vi "labviewRT_sm_example.vi"() -> ()   [LabVIEW 2020]
uses:
  lib/labviewRT-EPICS/sm bool read and increment.vi
  lib/labviewRT-EPICS/sm double read and increment.vi
  lib/labviewRT-EPICS/sm single read and increment.vi
  lib/labviewRT-EPICS/sm i64 read and increment.vi
  lib/labviewRT-EPICS/sm i32 read and increment.vi
  lib/labviewRT-EPICS/sm i16 read and increment.vi
  lib/labviewRT-EPICS/sm i8 read and increment.vi
  lib/labviewRT-EPICS/sm u64 read and increment.vi
  lib/labviewRT-EPICS/sm u32 read and increment.vi
  lib/labviewRT-EPICS/sm u16 read and increment.vi
  lib/labviewRT-EPICS/sm u8 read and increment.vi
  lib/labviewRT-EPICS/sm double write and increment.vi
  lib/labviewRT-EPICS/sm single write and increment.vi
  lib/labviewRT-EPICS/sm i64 write and increment.vi
  lib/labviewRT-EPICS/sm i32 write and increment.vi
  lib/labviewRT-EPICS/sm i16 write and increment.vi
  lib/labviewRT-EPICS/sm i8 write and increment.vi
  lib/labviewRT-EPICS/sm u64 write and increment.vi
  lib/labviewRT-EPICS/sm u32 write and increment.vi
  lib/labviewRT-EPICS/sm u16 write and increment.vi
  lib/labviewRT-EPICS/sm u8 write and increment.vi
  lib/labviewRT-EPICS/sm bool write and increment.vi
  lib/labviewRT-EPICS/linuxSharedMemory.lvlib
panel:
  in  "Boolean in":bool
  in  "U8":u8
  in  "U16":u16
  in  "U32":u32
  in  "U64":u64
  in  "I8":i8
  in  "I16":i16
  in  "I32":i32
  in  "I64":i64
  in  "Single":sgl format="%#_64g"
  in  "double":dbl format="%#_64g"
  out "U8":u8
  out "U16":u16
  out "U32":u32
  out "U64":u64
  out "I8":i8
  out "I16":i16
  out "I32":i32
  out "I64":i64
  out "Single":sgl format="%#_64g"
  out "double":dbl format="%#_64g"
  out "Boolean":bool
  in  "stop":bool
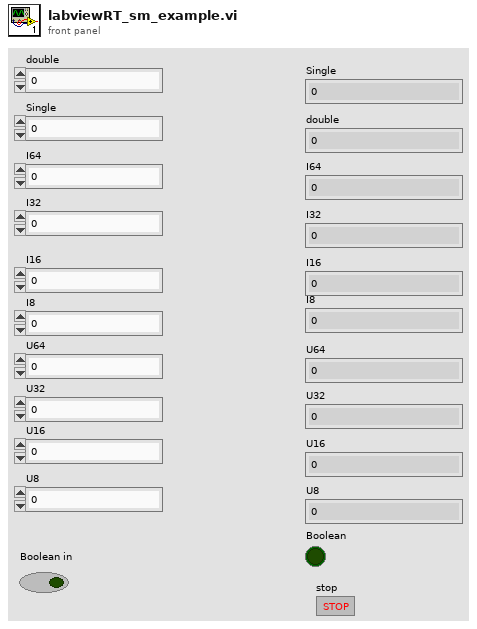
[diagram p1: front panel]
types:
  T1 = typedef "linuxSharedMemory.lvlib/sm_cluster.ctl" = cluster{"rt list":string, "error (no error)":errorcluster, "pointer":u64, "upper bound ptr":u64}
  T2 = typedef "Linux RT IPC.Shared Memory.lvlib/reference.ctl" = refnum<data-value>
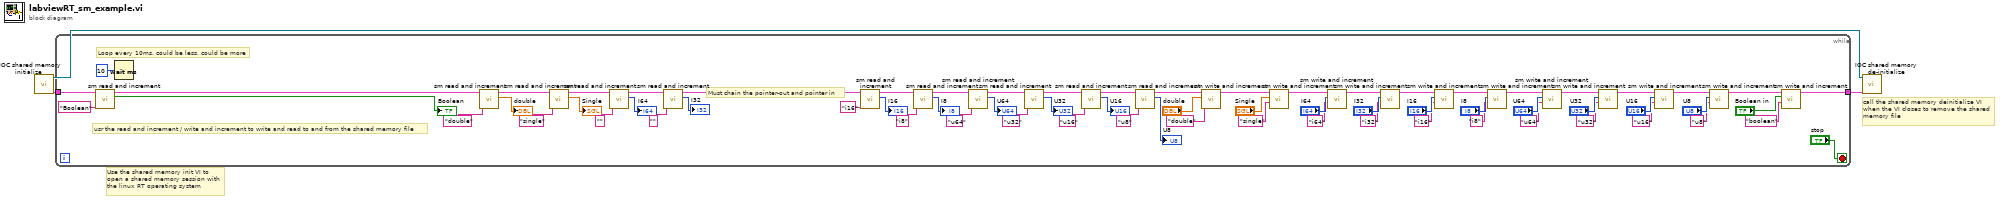
[diagram p0: block diagram]
diagram:
  # "call the shared memory deinitialize VI \nwhen the VI closes to remove the shared\nmemory file"
  # "Use the shared memory init VI to \nopen a shared memory session with\nthe linux RT operating system"
  n1 = call "IOC shared memory initialize.vi"() -> ("Shared memory cluster"=w2:T1, "shared memory class"=w3:T2)  [unwired: 10 in]
  n2 = while {
    tunnel: w2 -> [w27]
    tunnel: [w26] -> w1
    stop <- "stop" stop-if-true
    # "usr the read and increment / write and increment to write and read to and from the shared memory file"
    # "Must chain the pointer-out and pointer in"
    # "Loop every 10ms, could be less, could be more"
    n3 = call-poly "sm read and increment.vi"("Identifier"="Boolean", "Shared memory cluster input"=w27) -> ("Bool out"=→"Boolean":bool, "Shared memory cluster output"=w70:T1)  [unwired: 8 in]
    n4 = Wait (ms)(milliseconds to wait=10) -> ()  [unwired: 1 out]
    n5 = call-poly "sm read and increment.vi"("Identifier"="double", "Shared memory cluster input"=w70) -> ("Value out"=→"double":dbl, "Shared memory cluster output"=w69:T1)  [unwired: 8 in]
    n6 = call-poly "sm read and increment.vi"("Identifier"="single", "Shared memory cluster input"=w69) -> ("Value out"=→"Single":sgl, "Shared memory cluster output"=w68:T1)  [unwired: 8 in]
    n7 = call-poly "sm read and increment.vi"("Identifier"="", "Shared memory cluster input"=w68) -> ("Value out"=→"I64":i64, "Shared memory cluster output"=w67:T1)  [unwired: 8 in]
    n8 = call-poly "sm read and increment.vi"("Identifier"="", "Shared memory cluster input"=w67) -> ("Value out"=→"I32":i32, "Shared memory cluster output"=w66:T1)  [unwired: 8 in]
    n9 = call-poly "sm read and increment.vi"("Identifier"="i16", "Shared memory cluster input"=w66) -> ("Value out"=→"I16":i16, "Shared memory cluster output"=w65:T1)  [unwired: 8 in]
    n10 = call-poly "sm read and increment.vi"("Identifier"="i8", "Shared memory cluster input"=w65) -> ("Value out"=→"I8":i8, "Shared memory cluster output"=w64:T1)  [unwired: 8 in]
    n11 = call-poly "sm read and increment.vi"("Identifier"="u64", "Shared memory cluster input"=w64) -> ("Value out"=→"U64":u64, "Shared memory cluster output"=w63:T1)  [unwired: 8 in]
    n12 = call-poly "sm read and increment.vi"("Identifier"="u32", "Shared memory cluster input"=w63) -> ("Value out"=→"U32":u32, "Shared memory cluster output"=w61:T1)  [unwired: 8 in]
    n13 = call-poly "sm read and increment.vi"("Identifier"="u16", "Shared memory cluster input"=w61) -> ("Value out"=→"U16":u16, "Shared memory cluster output"=w62:T1)  [unwired: 8 in]
    n14 = call-poly "sm read and increment.vi"("Identifier"="u8", "Shared memory cluster input"=w62) -> ("Value out"=→"U8":u8, "Shared memory cluster output"=w48:T1)  [unwired: 8 in]
    n15 = call-poly "sm write and increment.vi"("Identifier"="double", "value in"="double", "Shared memory cluster input"=w48) -> ("Shared memory cluster output"=w47:T1)  [unwired: 8 in]
    n16 = call-poly "sm write and increment.vi"("Identifier"="single", "value in"="Single", "Shared memory cluster input"=w47) -> ("Shared memory cluster output"=w46:T1)  [unwired: 8 in]
    n17 = call-poly "sm write and increment.vi"("Identifier"="i64", "value in"="I64", "Shared memory cluster input"=w46) -> ("Shared memory cluster output"=w45:T1)  [unwired: 8 in]
    n18 = call-poly "sm write and increment.vi"("Identifier"="i32", "value in"="I32", "Shared memory cluster input"=w45) -> ("Shared memory cluster output"=w44:T1)  [unwired: 8 in]
    n19 = call-poly "sm write and increment.vi"("Identifier"="i16", "value in"="I16", "Shared memory cluster input"=w44) -> ("Shared memory cluster output"=w43:T1)  [unwired: 8 in]
    n20 = call-poly "sm write and increment.vi"("Identifier"="i8", "value in"="I8", "Shared memory cluster input"=w43) -> ("Shared memory cluster output"=w42:T1)  [unwired: 8 in]
    n21 = call-poly "sm write and increment.vi"("Identifier"="u64", "value in"="U64", "Shared memory cluster input"=w42) -> ("Shared memory cluster output"=w41:T1)  [unwired: 8 in]
    n22 = call-poly "sm write and increment.vi"("Identifier"="u32", "value in"="U32", "Shared memory cluster input"=w41) -> ("Shared memory cluster output"=w40:T1)  [unwired: 8 in]
    n23 = call-poly "sm write and increment.vi"("Identifier"="u16", "value in"="U16", "Shared memory cluster input"=w40) -> ("Shared memory cluster output"=w39:T1)  [unwired: 8 in]
    n24 = call-poly "sm write and increment.vi"("Identifier"="u8", "value in"="U8", "Shared memory cluster input"=w39) -> ("Shared memory cluster output"=w38:T1)  [unwired: 8 in]
    n25 = call-poly "sm write and increment.vi"("Identifier"="boolean", "value in"="Boolean in", "Shared memory cluster input"=w38) -> ("Shared memory cluster output"=w26:T1)  [unwired: 8 in]
  }
  n26 = call "IOC shared memory de-initialize.vi"("shared memory in"=w3, "Shared memory cluster"=w1) -> ()  [unwired: 9 in]
